vi "_storageSetDaqmxChannelProp.vi"(4 "Enum values":string[](array[string]), 6 "Channel Index":i32, 7 "Value":refnum<k21>, 8 "error in (no error)":errorcluster, 9 "Property name":string, 10 "Property source":string, 11 "storage refnum":refnum<k20>) -> (0 "error out":errorcluster, 3 "dup storage refnum":refnum<k20>)   [LabVIEW 2020]
uses:
  <vilib>/Platform/storage/Storage.llb/Set Property (I32).vi
  <vilib>/Platform/storage/Storage.llb/Set Property (DBL).vi
  <vilib>/Platform/storage/Storage.llb/Set Property (String).vi
  <vilib>/Platform/storage/Storage.llb/Set Property (Time Stamp).vi
  <vilib>/Utility/error.llb/whitespace.ctl
  <resource>/objmgr/daqmx.rc
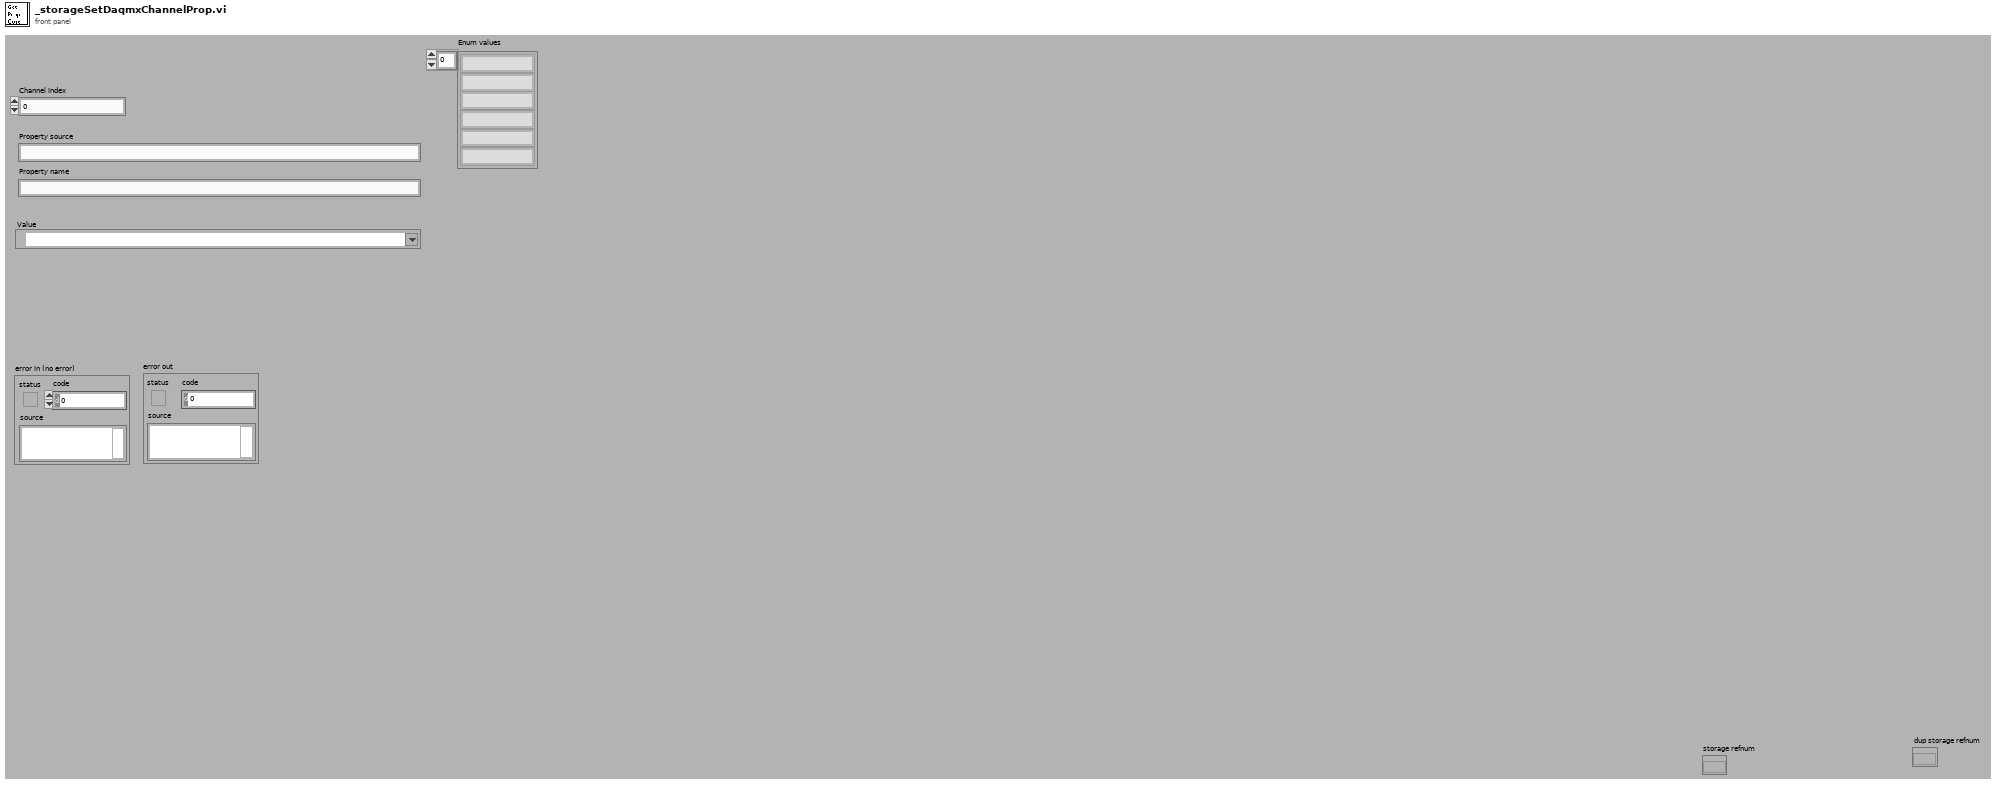
[diagram p1: front panel]
types:
  T1 = typedef "whitespace.ctl" = u16
  T2 = typedef "ex_TdmProperty.ctl" = cluster{"Name":string, "Type":T3, "Value":variant}
  T3 = typedef "usiDataType.ctl" = enum16{"eNoTypeUsi", "eInt8Usi", "eInt16Usi", "eInt32Usi", "eInt64Usi", "eUInt8Usi", "eUInt16Usi", "eUInt32Usi", "eUInt64Usi", "eFloat32Usi", "eFloat64Usi", "- 0", "- 1", "- 2", "- 3", "- 4", "- 5", "- 6", "- 7", "- 8", "- 9", "eString8Usi", "eString16Usi", "eStringUsi", "eEnumUsi", "- 10", "- 11", "- 12", "- 13", "- 14", "eTimeUsi", "- 15", "- 16", "- 17", "- 18", "- 19", "- 20", "- 21", "- 22", "- 23", "eInstanceUsi", "eStoreUsi"}
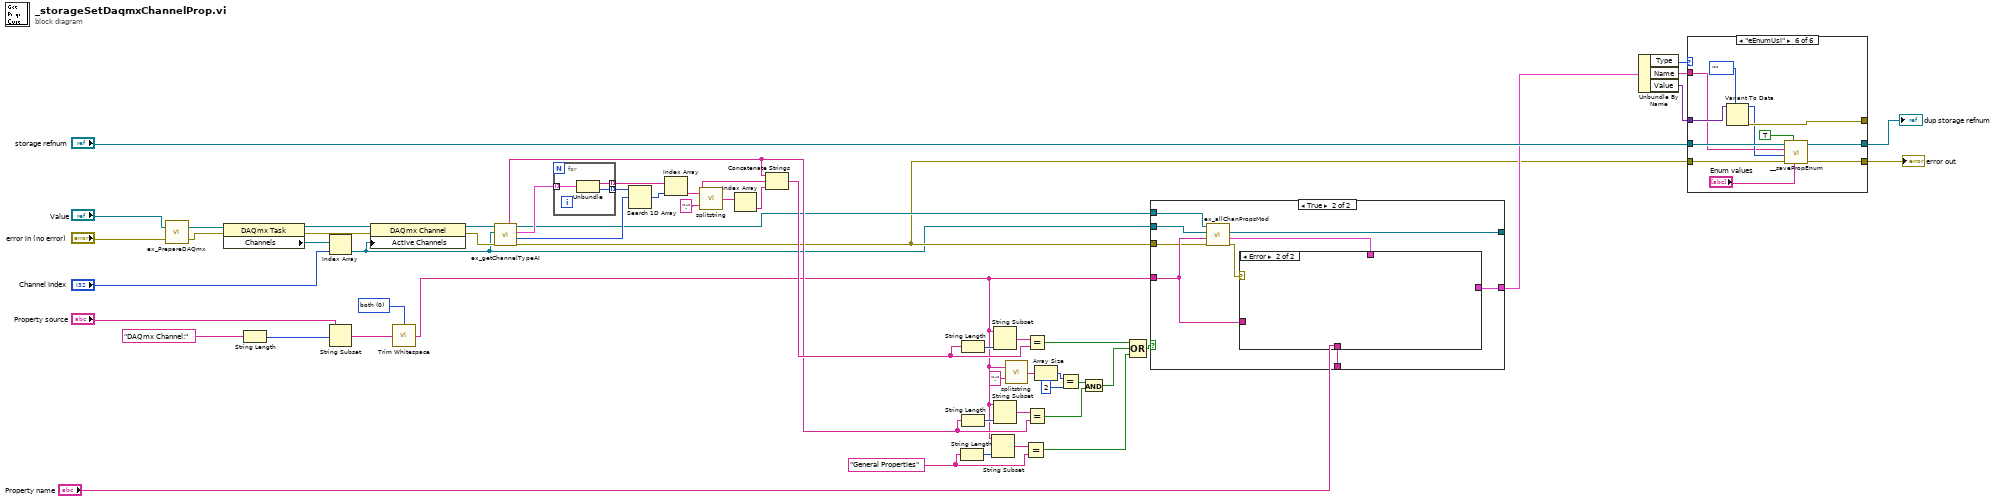
[diagram p0: block diagram]
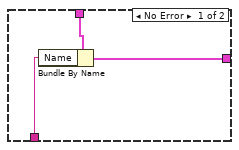
[diagram p3: hidden frame]
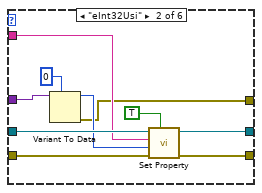
[diagram p5: hidden frame]
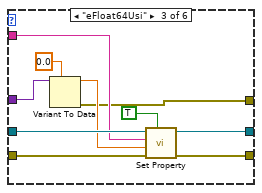
[diagram p6: hidden frame]
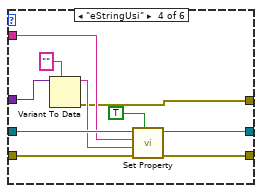
[diagram p7: hidden frame]
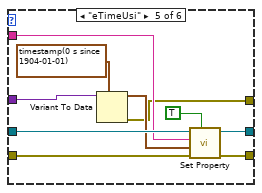
[diagram p8: hidden frame]
diagram:
  w7 = T1 0 items=["both", "start of string", "end of string"] ("location (both)")
  w33 = "General Properties" ("channel type")
  w40 = ":" ("search string/char (-)")
  n1 = call <vilib>:"ex_PrepareDAQmx.vi"("error in"="error in (no error)", "task/channels in"="Value") -> ("error out"=w50:errorcluster, "task out"=w51:refnum<k21>)
  n2 = property class="DAQmx Task"(reference=w51, error in=w50) -> (reference out=w55:refnum<k21>, error out=w54:errorcluster, "Channels"=w49:refnum<k21>[])
  n3 = String Length(string="DAQmx Channel:" ("search string/char (-)")) -> (length=w2:i32)
  n4 = Index Array(array=w49, index="Channel Index") -> (element=w1:refnum<k21>)
  n5 = String Subset(string="Property source", offset (0)=w2) -> (substring=w4:string)  [unwired: 1 in]
  n6 = property class="DAQmx Channel"(reference=w55, error in=w54, "Active Channels"=w1) -> (reference out=w35:refnum<k21>, error out=w38:errorcluster)
  n7 = call <vilib>:"Trim Whitespace.vi"("string"=w4, "location (both)"=w7) -> ("trimmed string"=w6:string)
  n8 = call <vilib>:"ex_getChannelTypeAI.vi"("error in (no error)"=w38, "DAQmx Global Channel"=w1, "task out"=w35) -> ("error out"=w9:errorcluster, "sub type"=w39:i32, "subsubtypes"=w44:cluster{"String":string, "Value":i32}[], "dup task"=w34:refnum<k21>, "channel type"=w36:string)  [unwired: 4 in]
  n9 = for {
    tunnel: w44 -> [w58] mode=indexing
    tunnel: [w57] -> w47 mode=indexing
    tunnel: [w56] -> w46 mode=indexing
    n10 = Unbundle(w58) -> ("String"=w56:string, "Value"=w57:i32)
  }
  n11 = Search 1D Array(1D array=w47, element=w39) -> (index of element=w45:i32)  [unwired: 1 in]
  n12 = Index Array(array=w46, index=w45) -> (element=w43:string)
  n13 = call <vilib>:"splitstring.vi"("search string/char (-)"=w40, "string"=w43) -> ("Array"=w37:string[])
  n14 = Index Array(array=w37) -> (element=w42:string)  [unwired: 1 in]
  n15 = Concatenate Strings(w36, w40, w42) -> (w41:string)
  n16 = String Length(string=w33) -> (length=w13:i32)
  n17 = String Length(string=w41) -> (length=w26:i32)
  n18 = String Length(string=w36) -> (length=w17:i32)
  n19 = String Subset(string=w6, length (rest)=w13) -> (substring=w12:string)  [unwired: 1 in]
  n20 = String Subset(string=w6, length (rest)=w26) -> (substring=w24:string)  [unwired: 1 in]
  n21 = String Subset(string=w6, length (rest)=w17) -> (substring=w18:string)  [unwired: 1 in]
  n22 = call <vilib>:"splitstring.vi"("search string/char (-)"=":", "string"=w6) -> ("Array"=w23:string[])
  n23 = Equal?(x=w12, y=w33) -> (x = y?=w11:bool)
  n24 = Equal?(x=w24, y=w41) -> (x = y?=w21:bool)
  n25 = Equal?(x=w18, y=w36) -> (x = y?=w15:bool)
  n26 = Array Size(array=w23) -> (size(s)=w22:i32)
  n27 = Equal?(x=w22, y=2) -> (x = y?=w16:bool)
  n28 = And(x=w16, y=w15) -> (x .and. y?=w14:bool)
  n29 = Compound Arithmetic op=OR(w21, w14, w11) -> (w20:bool)
  n30 = case shown="True" w20 {
    tunnel: w1 -> [w59 w68]
    tunnel: [w59 w67] -> _
    tunnel: w6 -> [_ w64]
    tunnel: w9 -> [_ w63]
    tunnel: w34 -> [_ w62]
    tunnel: "Property name" -> [_ w61]
    tunnel: [_ w60] -> w10
    frame False {
    }
    frame True {
      n31 = call <vilib>:"ex_allChanPropsMod.vi"("error in (no error)"=w63, "propertySource"=w64, "DAQmx Channel"=w68, "DAQmx Task"=w62) -> ("error out"=w65:errorcluster, "TDM Property"=w66:T2, "dup DAQmx Channel"=w67:refnum<k21>)  [unwired: 1 in]
      n32 = case shown="Error" w65 {
        tunnel: w66 -> [w71 _]
        tunnel: w64 -> [_ _]
        tunnel: w61 -> [w70 _]
        tunnel: [w69 _] -> w60
        frame No Error {
          n33 = Bundle By Name(cluster=w71, "Name"=w70) -> (w69:T2)
        }
        frame Error {
        }
      }
    }
  }
  n34 = Unbundle By Name(w10) -> ("Type"=w30:T3, "Name"=w31:string, "Value"=w32:variant)
  n35 = case shown="\"eEnumUsi\"" w30 {
    tunnel: w9 -> [w73 w83 w93 w103 w113 w122]
    tunnel: "storage refnum" -> [w72 w81 w91 w101 w111 w118]
    tunnel: [w73 w80 w90 w100 w110 w121] -> w8
    tunnel: w31 -> [_ w76 w89 w99 w109 w116]
    tunnel: w32 -> [_ w79 w88 w98 w108 w124]
    tunnel: [w72 w75 w85 w95 w105 w120] -> w28
    tunnel: [_ w74 w84 w94 w104 w119] -> _
    frame "eNoTypeUsi", Default {
    }
    frame "eInt32Usi" {
      n36 = Variant To Data(type=0, Variant=w79) -> (data=w77:i32, error out=w74:errorcluster)  [unwired: 1 in]
      n37 = call-poly <vilib>:"Set Property.vi"("Create if not found (no:F)"=TRUE, "error in (no error)"=w83, "Value"=w77, "Property name"=w76, "storage refnum"=w81) -> ("error out"=w80:errorcluster, "storage refnum out"=w75:refnum<k20>)  [unwired: 5 in]
    }
    frame "eFloat64Usi" {
      n38 = Variant To Data(type=0.0, Variant=w88) -> (data=w86:dbl, error out=w84:errorcluster)  [unwired: 1 in]
      n39 = call-poly <vilib>:"Set Property.vi"("Create if not found (no:F)"=TRUE, "error in (no error)"=w93, "Value"=w86, "Property name"=w89, "storage refnum"=w91) -> ("error out"=w90:errorcluster, "storage refnum out"=w85:refnum<k20>)  [unwired: 5 in]
    }
    frame "eStringUsi" {
      n40 = Variant To Data(type="", Variant=w98) -> (data=w96:string, error out=w94:errorcluster)  [unwired: 1 in]
      n41 = call-poly <vilib>:"Set Property.vi"("Create if not found (no:F)"=TRUE, "error in (no error)"=w103, "Value"=w96, "Property name"=w99, "storage refnum"=w101) -> ("error out"=w100:errorcluster, "storage refnum out"=w95:refnum<k20>)  [unwired: 5 in]
    }
    frame "eTimeUsi" {
      n42 = Variant To Data(type=timestamp(0 s since 1904-01-01), Variant=w108) -> (data=w107:timestamp, error out=w104:errorcluster)  [unwired: 1 in]
      n43 = call-poly <vilib>:"Set Property.vi"("Create if not found (no:F)"=TRUE, "error in (no error)"=w113, "Value"=w107, "Property name"=w109, "storage refnum"=w111) -> ("error out"=w110:errorcluster, "storage refnum out"=w105:refnum<k20>)  [unwired: 5 in]
    }
    frame "eEnumUsi" {
      n44 = Variant To Data(type=enum16{""}."", Variant=w124) -> (data=w117:enum16{""}, error out=w119:errorcluster)  [unwired: 1 in]
      n45 = call <vilib>:"__savePropEnum.vi"("Enum values"="Enum values", "User-defined property"=TRUE, "error in (no error)"=w122, "Value"=w117, "Property name"=w116, "storage refnum"=w118) -> ("error out"=w121:errorcluster, "dup storage refnum"=w120:refnum<k20>)  [unwired: 4 in]
    }
  }
  "error out" <- w8
  "dup storage refnum" <- w28
